vi "Prober_ChuckUpDown.vi"(8 "error in (no error)":errorcluster, 10 "Direction":enum16{"up", "down"}(ring), 11 "VeloxTeslaProbestation in":refnum<class "VeloxTeslaProbestation.lvclass">) -> (0 "error out":errorcluster, 2 "Chuck at CONTACT?":bool=TRUE, 3 "VeloxTeslaProbestation out":refnum<class "VeloxTeslaProbestation.lvclass">)   [LabVIEW 2018, in "VeloxTeslaProbestation.lvclass"]
uses:
  VeloxTeslaProbestation.lvclass
  Desktop/Kvasnicka/test_labview_library/Integration_toolkit_library/CascadeProbestation.lvlib
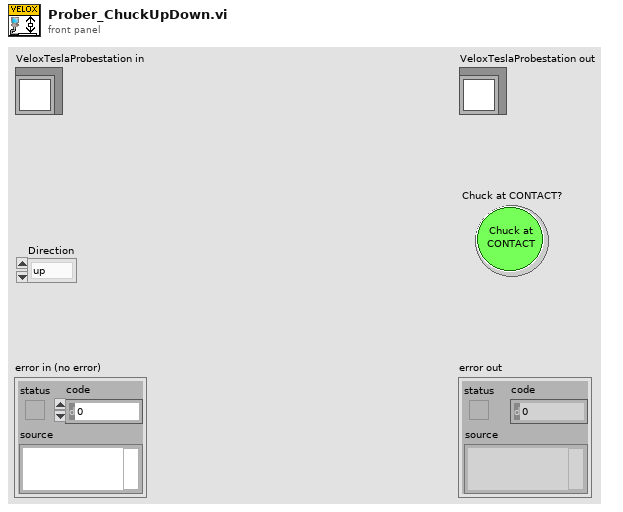
[diagram p1: front panel]
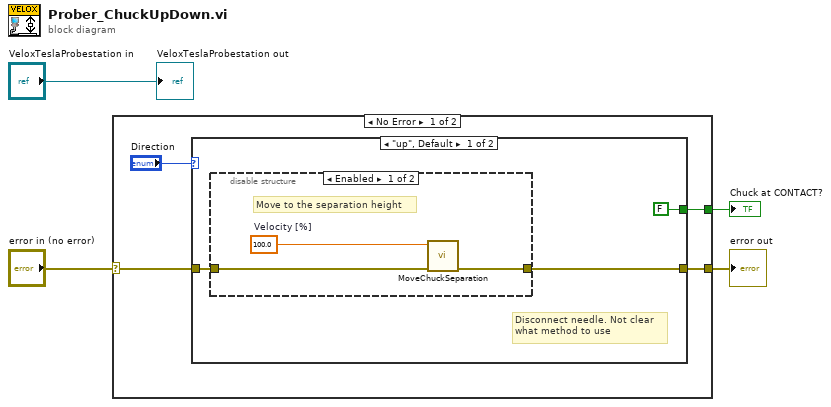
[diagram p0: block diagram]
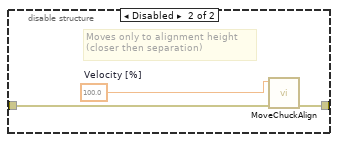
[diagram p2: hidden frame]
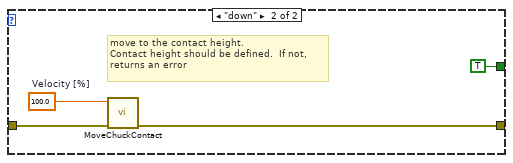
[diagram p3: hidden frame]
diagram:
  n1 = case shown="No Error" "error in (no error)" {
    selector: "error in (no error)" -> [w5 w22]
    tunnel: [w7 w22] -> w4
    tunnel: [w6 _] -> w3
    frame No Error {
      n2 = case shown="\"up\", Default" "Direction" {
        tunnel: w5 -> [w11 w20]
        tunnel: [w10 w19] -> w7
        tunnel: [FALSE ("Chuck at CONTACT?") TRUE ("Chuck at CONTACT?")] -> w6
        frame "up", Default {
          # "Disconnect needle. Not clear\nwhat method to use"
          n3 = disable-structure shown="Enabled" {
            disable-tunnel: w11 -> [w13 w17]
            disable-tunnel: [w12 w16] -> w10
            frame Enabled {
              w14 = 100.0  # Velocity [%]
              # "Move to the separation height"
              n4 = call "MoveChuckSeparation.vi"("Error In"=w13, "Velocity"=w14) -> ("Error Out"=w12:errorcluster)  [unwired: 8 in, 1 out]
            }
            frame Disabled {
              w15 = 100.0  # Velocity [%]
              # "Moves only to alignment height\n(closer then separation)"
              n5 = call "MoveChuckAlign.vi"("Error In"=w17, "Velocity"=w15) -> ("Error Out"=w16:errorcluster)  [unwired: 8 in, 1 out]
            }
          }
        }
        frame "down" {
          w21 = 100.0  # Velocity [%]
          # "move to the contact height.\nContact height should be defined.  If not,\nreturns an error"
          n6 = call "MoveChuckContact.vi"("Error In"=w20, "Velocity"=w21) -> ("Error Out"=w19:errorcluster)  [unwired: 8 in, 1 out]
        }
      }
    }
    frame Error {
    }
  }
  "error out" <- w4
  "Chuck at CONTACT?" <- w3
  "VeloxTeslaProbestation out" <- "VeloxTeslaProbestation in"
